vi "Verify Device is Present.vi"(8 "Error In":errorcluster, 11 "Serial Number in":string) -> (0 "Error Out":errorcluster, 3 "Present?":bool)   [LabVIEW 2018, in "ThorlabsLabJack.lvlib" / "ThorlabsLabJack.lvclass"]
uses:
  ThorlabsLabJack.lvclass
  C:/AME Test Engineering/LabVIEW/PPLs/Axis/DLLs/Thorlabs.MotionControl.DeviceManagerCLI.dll
  PPLs/Axis/DLLs/Thorlabs.MotionControl.DeviceManagerCLI.dll
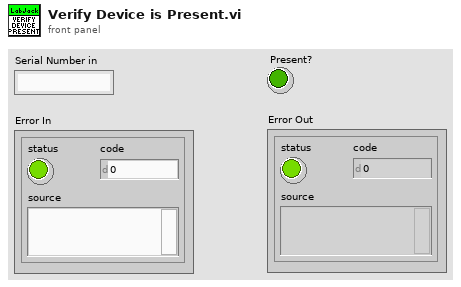
[diagram p1: front panel]
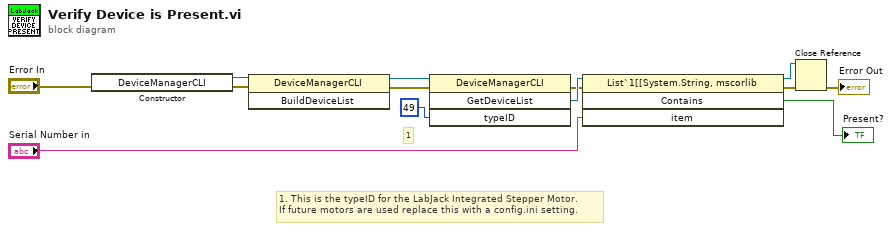
[diagram p0: block diagram]
diagram:
  # "1. This is the typeID for the LabJack Integrated Stepper Motor.\nIf future motors are used replace this with a config.ini setting."
  # "1"
  n1 = constructor class="DeviceManagerCLI"(error in="Error In") -> (reference out=w4:refnum<k24>, error out=w3:errorcluster)  [unwired: 2 in, 1 out]
  n2 = invoke class="DeviceManagerCLI" method="BuildDeviceList"(reference=w4, error in=w3) -> (reference out=w6:refnum<k24>, error out=w12:errorcluster)  [unwired: 1 in, 1 out]
  n3 = invoke class="DeviceManagerCLI" method="GetDeviceList"(reference=w6, error in=w12, "typeID"=49) -> (error out=w9:errorcluster, "GetDeviceList"=w10:refnum<k24>)  [unwired: 1 in, 2 out]
  n4 = invoke class="List`1[[System.String, mscorlib" method="Contains"(reference=w10, error in=w9, "item"="Serial Number in") -> (reference out=w7:refnum<k24>, error out=w8:errorcluster, "Contains"=→"Present?":bool)  [unwired: 1 in, 1 out]
  n5 = Close Reference(reference=w7, error in (no error)=w8) -> (error out=→"Error Out":errorcluster)
